vi "GetText.vi"(8 "error in":errorcluster, 11 "Engine in":refnum<class "CVT Engine Editor.lvclass">) -> (0 "error out":errorcluster, 1 "additional text":string, 2 "text":string, 3 "Engine out":refnum<class "CVT Engine Editor.lvclass">, 4 "glyph":string)   [LabVIEW 2013, in "CVT Engine Editor.lvclass"]
uses:
  CVT Engine Editor.lvclass
  <vilib>/NI/Tag Bus Data Framework/Configuration Editor/Classes/Engine Parent/Engine Parent Editor Node.lvclass
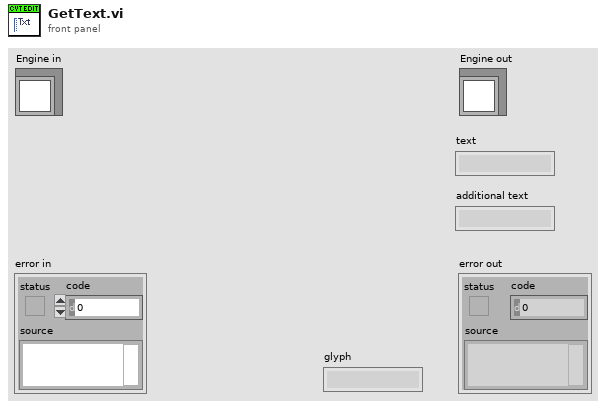
[diagram p1: front panel]
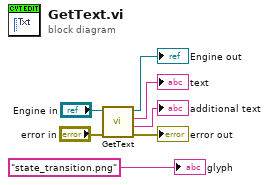
[diagram p0: block diagram]
diagram:
  n1 = call-parent "GetText.vi"("error in"="error in", "Engine in"="Engine in") -> ("error out"=→"error out":errorcluster, "additional text"=→"additional text":string, "text"=→"text":string, "Engine out"=→"Engine out":refnum<class "CVT Engine Editor.lvclass">)  [unwired: 5 in, 1 out]
  "glyph" <- "state_transition.png" ("Name")
